vi "RTS Find Base Filename.vi"(8 "Error In":errorcluster, 11 "Input name":string) -> (0 "Error Out":errorcluster, 4 "Base File Name":string)   [LabVIEW 2020]
uses:
  <vilib>/Utility/error.llb/whitespace.ctl
panel:
  out "No Match":bool
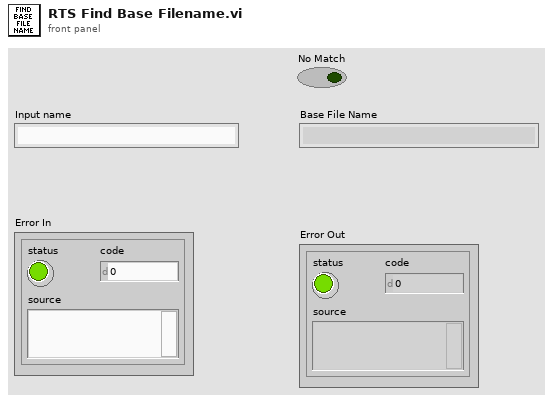
[diagram p1: front panel]
types:
  T1 = typedef "whitespace.ctl" = u16
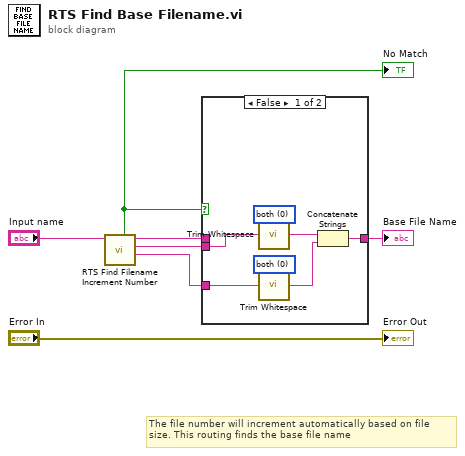
[diagram p0: block diagram]
diagram:
  # "The file number will increment automatically based on file\nsize. This routing finds the base file name"
  n1 = call "RTS Find Filename Increment Number.vi"("Input name in"="Input name") -> ("After Find"=w1:string, "Before Find"=w5:string, "Full Input Name"=w6:string, "No Match"=w2:bool)  [unwired: 7 in]
  "No Match" <- w2
  n2 = case shown="False" w2 {
    tunnel: w5 -> [w10 _]
    tunnel: w1 -> [w9 _]
    tunnel: w6 -> [_ w15]
    tunnel: [w8 w15] -> w7
    frame False {
      w13 = T1 0 items=["both", "start of string", "end of string"] ("location (both)")
      w12 = T1 0 items=["both", "start of string", "end of string"] ("location (both)")
      n3 = call <vilib>:"Trim Whitespace.vi"("string"=w10, "location (both)"=w12) -> ("trimmed string"=w11:string)
      n4 = call <vilib>:"Trim Whitespace.vi"("string"=w9, "location (both)"=w13) -> ("trimmed string"=w14:string)
      n5 = Concatenate Strings(w11, w14) -> (w8:string)
    }
    frame True {
    }
  }
  "Base File Name" <- w7
  "Error Out" <- "Error In"
